vi "FPGA_Main2.vi"() -> ()   [LabVIEW 2018]
uses:
  <vilib>/Platform/TimedLoop/XDataNode/timing_clust.ctl
  <vilib>/Platform/TimedLoop/XDataNode/nitl_modes.ctl
  <vilib>/Platform/TimedLoop/XDataNode/wakeup.ctl
  <vilib>/rvi/Emulation/niFpgaGetClockAttributes.vi
  <vilib>/rvi/Emulation/niFpgaSctlEmulationGetInTimedLoop.vi
  <vilib>/rvi/Emulation/niFpgaEmulationReportErrorSimple.vi
  <vilib>/rvi/Emulation/niFpgaProcessEmulError.vi
  <vilib>/rvi/Emulation/niFpgaCriticalErrorInLSC.vi
  <vilib>/rvi/eio/common/nirviEmuTemplateMethod_errors.vi
  <vilib>/eio/EIONode/EIONode.xnode
  <vilib>/platform/TimedLoop/XDataNode/XDataNode.xnode
  <vilib>/Platform/TimedLoop/XDataNode/XDNodeRunTimeDep.lvlib
panel:
  in  "speed step":u32
  in  "pwm_val":u32=1000
  in  "delaya":u32=10
  in  "gap min":i16
  in  "gap max":i16
  out "off_track":bool
  out "scaled_speed":i16
  in  "delay_pwm_us":u32=100
  in  "sp_scale":i16=40
  in  "sp_max_limit":u16=600
  in  "sp_min_limit":u16=400
  out "Waveform Chart":i16(graph)
  out "gap_pos":i16=-1
  out "speed":i16
  in  "dt_pwm_ms":u32=300 caption="Count(uSec)"
  out "busy":bool
  in  "dt_m_us":u32=1 caption="delay_M_ms"
  in  "setpoint":i16
  in  "stop_band":i16=4
  in  "inv":bool=TRUE
  out "AI0":u16=1344
  out "dAI":i16=8
  out "backward":bool
  out "pos":i16=1241
  out "err cnt":i16
  in  "reset":bool
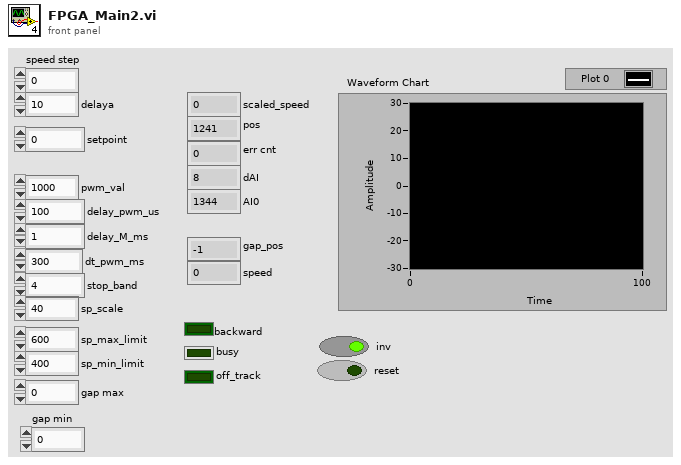
[diagram p1: front panel]
types:
  T1 = typedef "XDNodeRunTimeDep.lvlib/timing_clust.ctl" = cluster{"Expected End [f-1]":u64, "Actual End [f-1]":u64, "Finished Late? [f-1]":bool, "Expected End [i-1]":u64, "Actual End [i-1]":u64, "Finished Late? [i-1]":bool, "Expected Start [i]":u64, "Actual Start [i]":u64, "Expected Start [f]":u64, "Actual Start [f]":u64, "Source Name":string, "Structure Name":string, "Period":i64, "Deadline":i64, "Offset":i64, "Start":i64, "Priority":i32, "Timeout":i32, "Mode":T2, "Wakeup Reason":T3, "Error":errorcluster, "Source Type":string, "Secondary Source Type":string, "Global End Time":u64, "Global Start Time":u64, "Frame Duration":u64, "Iteration Duration":u64, "Assigned CPU":i32, "I/O Scan Engine Mode":u32}
  T2 = typedef "XDNodeRunTimeDep.lvlib/nitl_modes.ctl" = enum32{"No Change", "Process missed periods, maintain original phase", "Discard missed periods, maintain original phase", "Process missed periods, ignore original phase", "Discard missed periods, ignore original phase"}
  T3 = typedef "XDNodeRunTimeDep.lvlib/wakeup.ctl" = enum32{"Normal", "Aborted", "Asynchronous wakeup", "Timing source error", "Timed loop error", "Timeout"}
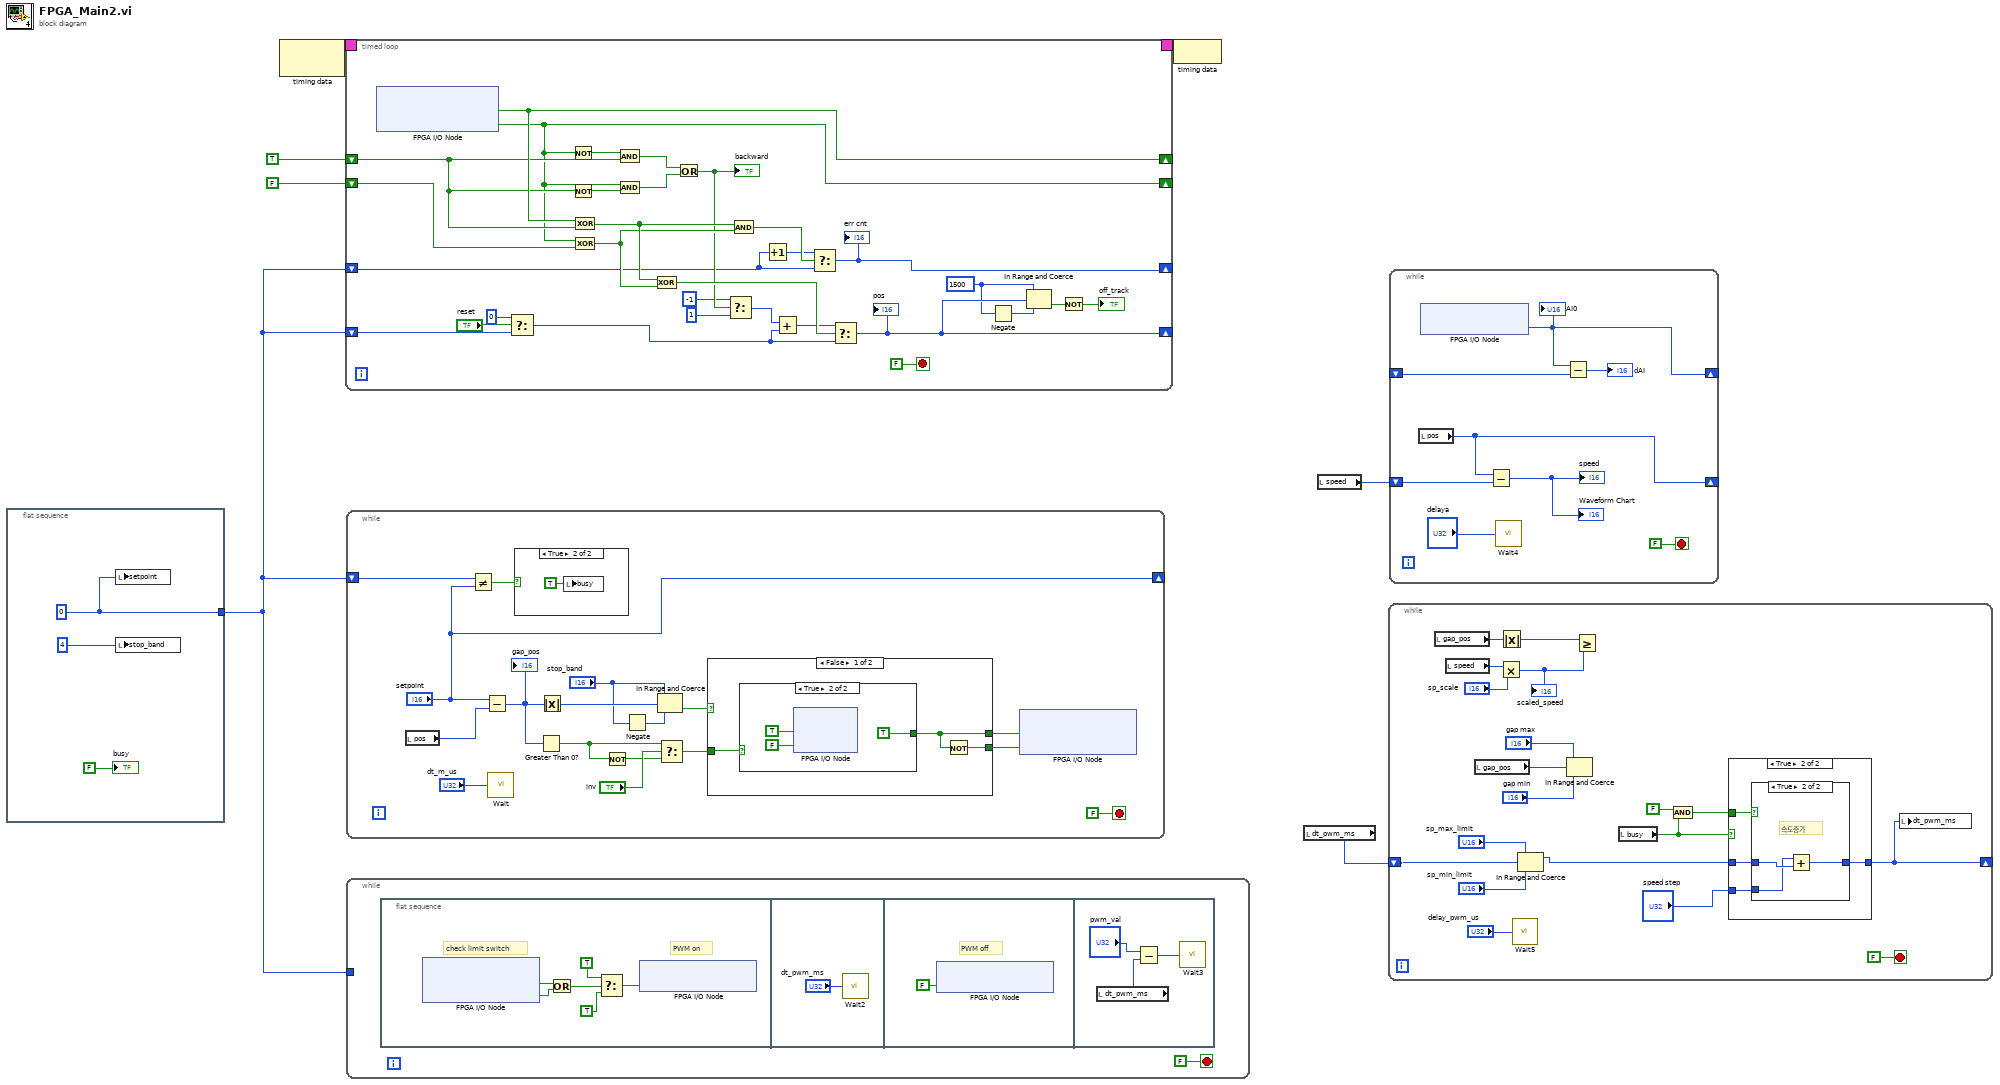
[diagram p0: block diagram]
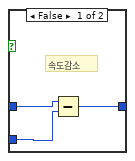
[diagram p3: hidden frame]
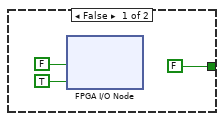
[diagram p5: hidden frame]
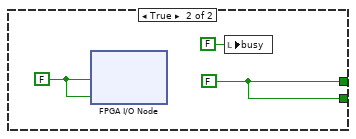
[diagram p6: hidden frame]
diagram:
  n1 = flat-sequence {
    tunnel: [w9] -> w3
    frame #0 {
      w9 = i16 0
      n2 = local write "setpoint"(w9) -> ()
      n3 = local write "stop_band"(i16 4 ("dead band")) -> ()
      "busy" <- FALSE ("status")
    }
  }
  n4 = node-c288() -> (w7:T1)  [unwired: 1 in]
  n5 = timed-loop {
    timing: w7 -> [_]
    timing-out: [_] -> w6
    shift-right: [w35] -> _
    shift-left: TRUE ("ConnectorA/DIO11") -> [w34]
    shift-right: [w33] -> _
    shift-left: FALSE ("ConnectorA/DIO12") -> [w32]
    shift-right: [w15] -> _
    shift-left: w3 -> [w18]
    shift-right: [w20] -> _
    shift-left: w3 -> [w21]
    stop <- FALSE stop-if-true
    w11 = i16 1500 ("upper limit")
    n6 = xnode "FPGA I/O Node"() -> ("ConnectorA/DIO11"=w35:bool, "ConnectorA/DIO12"=w33:bool)  [unwired: 2 in, 2 out]
    n7 = Select(t=i16 0, s="reset", f=w18) -> (s? t:f=w16:i16)
    n8 = Not(x=w33) -> (.not. x?=w39:bool)
    n9 = Not(x=w34) -> (.not. x?=w38:bool)
    n10 = Exclusive Or(1:w34, 2:w35) -> (0:w31:bool)
    n11 = Exclusive Or(1:w32, 2:w33) -> (0:w30:bool)
    n12 = And(x=w39, y=w34) -> (x .and. y?=w36:bool)
    n13 = And(x=w33, y=w38) -> (x .and. y?=w37:bool)
    n14 = Exclusive Or(1:w30, 2:w31) -> (0:w29:bool)
    n15 = Or(x=w36, y=w37) -> (x .or. y?=w28:bool)
    "backward" <- w28
    n16 = Select(t=i16 -1, s=w28, f=i16 1) -> (s? t:f=w25:i16)
    n17 = And(x=w31, y=w30) -> (x .and. y?=w23:bool)
    n18 = Increment(x=w21) -> (x+1=w22:i16)
    n19 = Add(x=w25, y=w16) -> (x+y=w24:i16)
    n20 = Select(t=w22, s=w23, f=w21) -> (s? t:f=w20:i16)
    "err cnt" <- w20
    n21 = Select(t=w24, s=w29, f=w16) -> (s? t:f=w15:i16)
    "pos" <- w15
    n22 = Negate(x=w11) -> (-x=w12:i16)
    n23 = In Range and Coerce(upper limit=w11, x=w15, lower limit=w12) -> (In Range?=w14:bool)  [unwired: 1 out]
    n24 = Not(x=w14) -> (.not. x?=→"off_track":bool)
  }
  n25 = while {
    shift-right: ["setpoint"] -> _
    shift-left: w3 -> [w44]
    stop <- FALSE stop-if-true
    n26 = local read "pos"() -> (w55:i16)
    n27 = Not Equal?(x=w44, y="setpoint") -> (x != y?=w43:bool)
    n28 = Subtract(x="setpoint", y=w55) -> (x-y=w46:i16)
    "gap_pos" <- w46
    n29 = call "Wait"("Count(uSec)"="dt_m_us") -> ()  [unwired: 1 out]
    n30 = case shown="True" w43 {
      frame False {
      }
      frame True {
        n31 = local write "busy"(TRUE ("busy")) -> ()
      }
    }
    n32 = Greater Than 0?(x=w46) -> (x > 0?=w48:bool)
    n33 = Absolute Value(x=w46) -> (abs(x)=w54:i16)
    n34 = Not(x=w48) -> (.not. x?=w49:bool)
    n35 = Negate(x="stop_band") -> (-x=w53:i16)
    n36 = In Range and Coerce(upper limit="stop_band", x=w54, lower limit=w53) -> (In Range?=w51:bool)  [unwired: 1 out]
    n37 = Select(t=w48, s="inv", f=w49) -> (s? t:f=w47:bool)
    n38 = case shown="False" w51 {
      tunnel: [w63 w72] -> w57
      tunnel: [w62 w72] -> w56
      tunnel: w47 -> [w61 _]
      frame False {
        n39 = case shown="True" w61 {
          tunnel: [FALSE ("dir") TRUE ("dir")] -> w62
          frame False {
            n40 = xnode "FPGA I/O Node"("LED0"=FALSE, "LED1"=TRUE) -> ()  [unwired: 2 in, 2 out]
          }
          frame True {
            n41 = xnode "FPGA I/O Node"("LED0"=TRUE, "LED1"=FALSE) -> ()  [unwired: 2 in, 2 out]
          }
        }
        n42 = Not(x=w62) -> (.not. x?=w63:bool)
      }
      frame True {
        w70 = FALSE ("LED0")
        w72 = FALSE ("dir")
        n43 = xnode "FPGA I/O Node"("LED0"=w70, "LED1"=w70) -> ()  [unwired: 2 in, 2 out]
        n44 = local write "busy"(FALSE ("busy")) -> ()
      }
    }
    n45 = xnode "FPGA I/O Node"("ConnectorA/DIO6"=w56, "ConnectorA/DIO5"=w57) -> ()  [unwired: 2 in, 2 out]
  }
  n46 = while {
    tunnel: w3 -> [_]
    stop <- FALSE stop-if-true
    n47 = flat-sequence {
      frame #0 {
        # "check limit switch"
        # "PWM on"
        n48 = xnode "FPGA I/O Node"() -> ("ConnectorA/DIO0"=w78:bool, "ConnectorA/DIO1"=w79:bool)  [unwired: 2 in, 2 out]
        n49 = Or(x=w78, y=w79) -> (x .or. y?=w77:bool)
        n50 = Select(t=TRUE, s=w77, f=TRUE ("ConnectorA/DIO8")) -> (s? t:f=w76:bool)
        n51 = xnode "FPGA I/O Node"("ConnectorA/DIO8"=w76) -> ()  [unwired: 1 in, 1 out]
      }
      frame #1 {
        n52 = call "Wait2"("Count(uSec)"="dt_pwm_ms") -> ()  [unwired: 1 out]
      }
      frame #2 {
        # "PWM off"
        n53 = xnode "FPGA I/O Node"("ConnectorA/DIO8"=FALSE) -> ()  [unwired: 1 in, 1 out]
      }
      frame #3 {
        n54 = local read "dt_pwm_ms"() -> (w84:u32)
        n55 = Subtract(x="pwm_val", y=w84) -> (x-y=w82:u32)
        n56 = call "Wait3"("Count(uSec)"=w82) -> ()  [unwired: 1 out]
      }
    }
  }
  n57 = node-c288(w6) -> ()
  n58 = local read "dt_pwm_ms"() -> (w2:u32)
  n59 = local read "speed"() -> (w1:i16)
  n60 = while {
    shift-right: [w94] -> _
    shift-left: w2 -> [w93]
    stop <- FALSE stop-if-true
    n61 = local read "gap_pos"() -> (w101:i16)
    n62 = local read "speed"() -> (w98:i16)
    n63 = local read "gap_pos"() -> (w90:i16)
    n64 = Multiply(x=w98, y="sp_scale") -> (x*y=w96:i16)
    "scaled_speed" <- w96
    n65 = Absolute Value(x=w101) -> (abs(x)=w99:i16)
    n66 = call "Wait5"("Count(uSec)"="delay_pwm_us") -> ()  [unwired: 1 out]
    n67 = In Range and Coerce(upper limit="sp_max_limit", x=w93, lower limit="sp_min_limit") -> (coerced(x)=w87:u32)  [unwired: 1 out]
    n68 = In Range and Coerce(upper limit="gap max", x=w90, lower limit="gap min") -> ()  [unwired: 2 out]
    n69 = Greater Or Equal?(x=w99, y=w96) -> ()  [unwired: 1 out]
    n70 = local read "busy"() -> (w86:bool)
    n71 = And(x=FALSE, y=w86) -> (x .and. y?=w100:bool)
    n72 = case shown="True" w86 {
      tunnel: [w104 w108] -> w94
      tunnel: w100 -> [_ w107]
      tunnel: w87 -> [w104 w106]
      tunnel: "speed step" -> [_ w105]
      frame False {
        # "속도유지"
      }
      frame True {
        n73 = case shown="True" w107 {
          tunnel: w106 -> [w110 w114]
          tunnel: [w111 w113] -> w108
          tunnel: w105 -> [w109 w112]
          frame False {
            # "속도감소"
            n74 = Subtract(x=w110, y=w109) -> (x-y=w111:u32)
          }
          frame True {
            # "속도증가"
            n75 = Add(x=w112, y=w114) -> (x+y=w113:u32)
          }
        }
      }
    }
    n76 = local write "dt_pwm_ms"(w94) -> ()
  }
  n77 = while {
    shift-right: [w120] -> _
    shift-left: w1 -> [w119]
    shift-right: [w116] -> _
    shift-left: _ -> [w117]
    stop <- FALSE stop-if-true
    n78 = local read "pos"() -> (w120:i16)
    n79 = xnode "FPGA I/O Node"() -> ("ConnectorA/AI0"=w116:u16)  [unwired: 1 in, 1 out]
    "AI0" <- w116
    n80 = Subtract(x=w120, y=w119) -> (x-y=→"speed" →"Waveform Chart":i16)
    n81 = call "Wait4"("Count(mSec)"="delaya") -> ()  [unwired: 1 out]
    n82 = Subtract(x=w116, y=w117) -> (x-y=→"dAI":u16)
  }
